vi "Single Loop QSM.vi"   [LabVIEW 2016, in "SLL QSM.lvlib"]
doc: "General Purpose Queue Based State Machine for Any Use Case (main application, module, pop up message etc)\n\n<b>Advantages:</b>\n1. No Need to Pass Queue References between Queue Driver VIs.\n2. This template can be safely used in multiple parallel running modules without any issues.\n3. This template can also be safely used even in cases where the VI is configured to be a Clone, where multiple \ninstances of the VI could be executing concurrently.\n\n<b>How to Use:</b>\n1. Add necessary items to the Main Cluster.\n2. Use the Polymorphic Queue Driver for doing any queue operations. There is no need to pass the queue driver\nreference, as the Queue Driver automatically infers the reference based on the VI instance from which it is called.\n3. Add any required user events in the \"Register Events\" case. Ignore if not needed.\n4. Use \"Sequences\" section for defining any list of state calls, which could be used in multiple places. \nEg: Initialize Sequence, might be needed if we need to any reinitialization."
uses:
  SLL QSM.lvlib
  <vilib>/Utility/error.llb/DialogType.ctl
  Queue Driver/Create Queue.vi
  Queue Driver/Enqueue an Item to Queue.vi
  Queue Driver/Dequeue Queue.vi
  Queue Driver/Enqueue N Items.vi
  Queue Driver/Flush Queue.vi
  Queue Driver/Release Queue.vi
types:
  T1 = typedef "DialogType.ctl" = u16
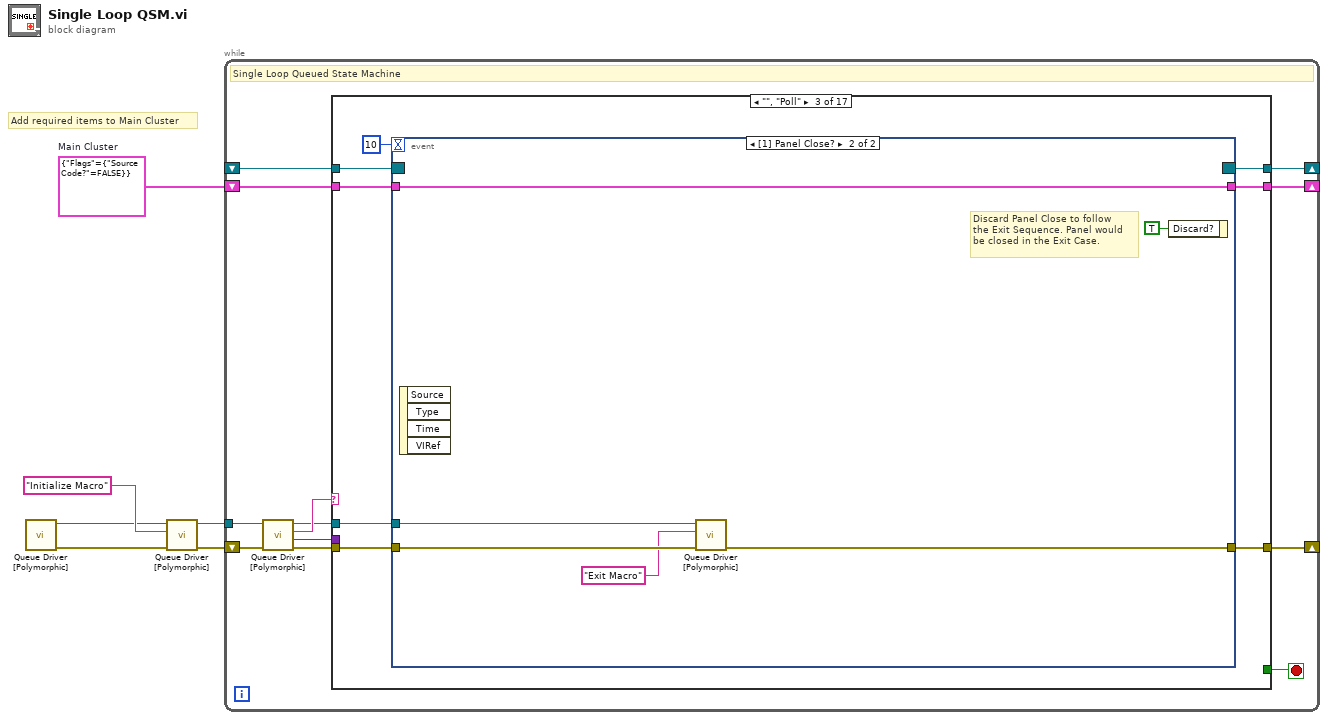
[diagram p0: block diagram]
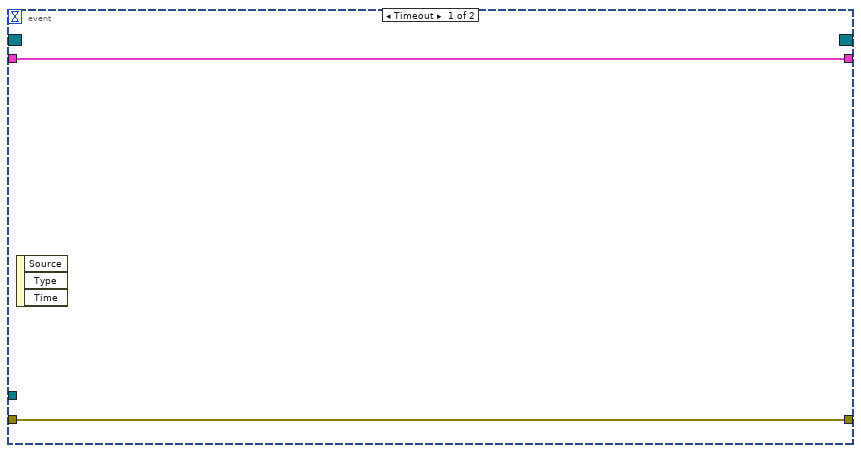
[diagram p4: hidden frame]
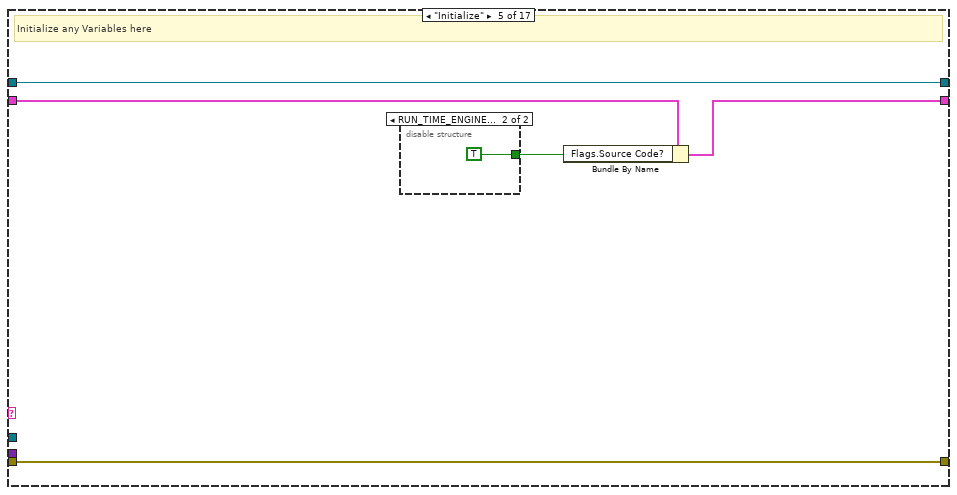
[diagram p6: hidden frame]
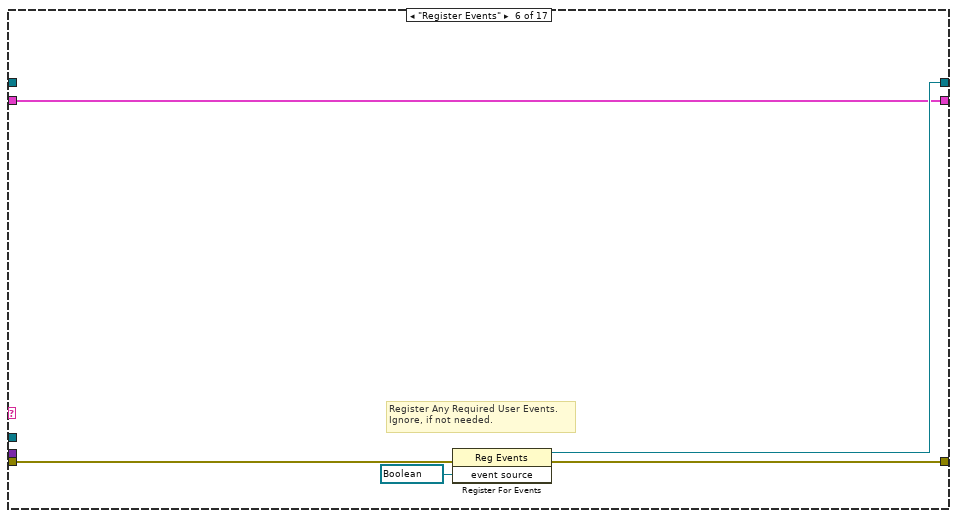
[diagram p8: hidden frame]
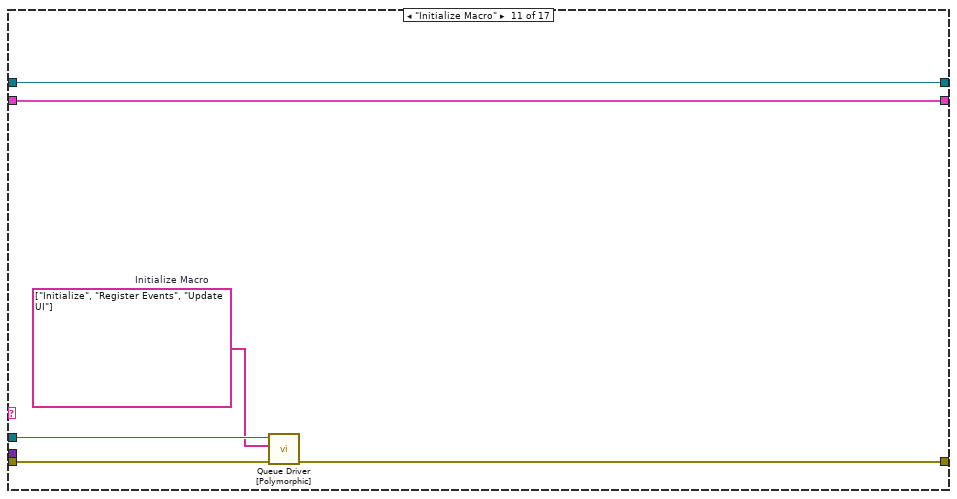
[diagram p13: hidden frame]
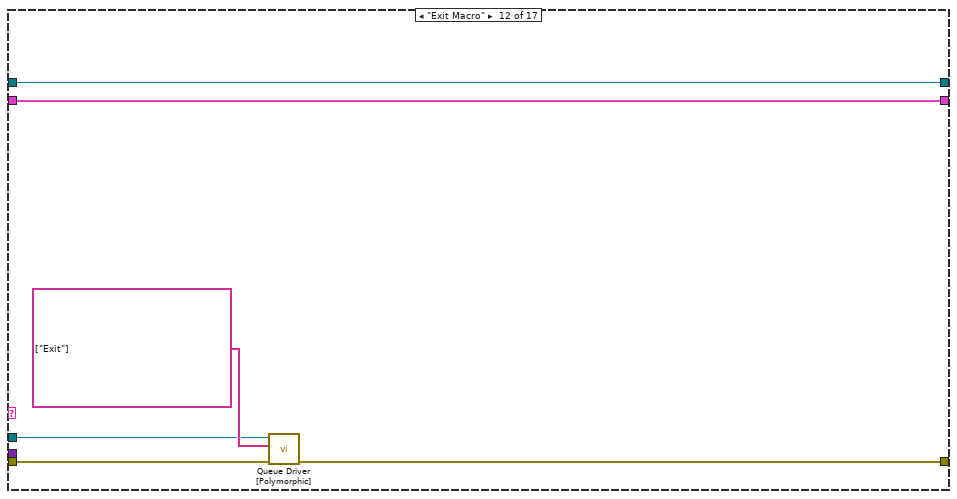
[diagram p14: hidden frame]
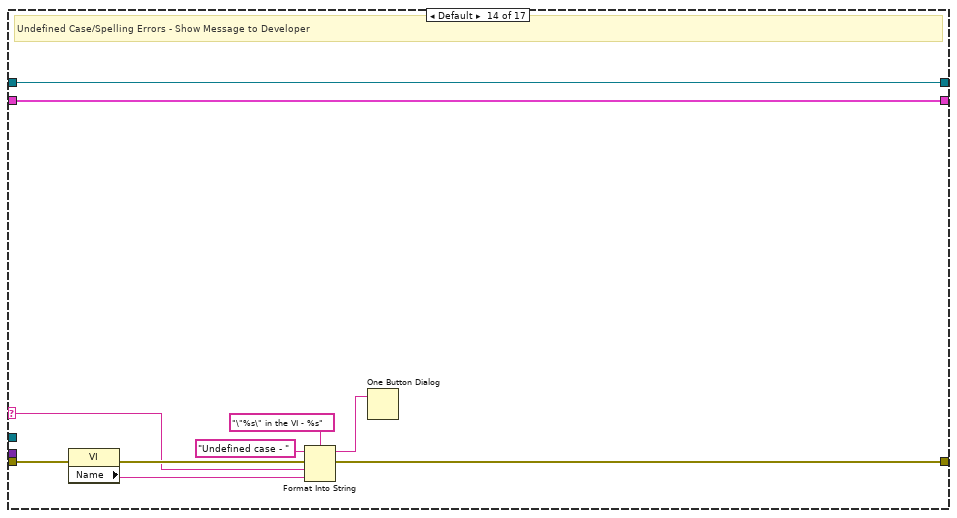
[diagram p16: hidden frame]
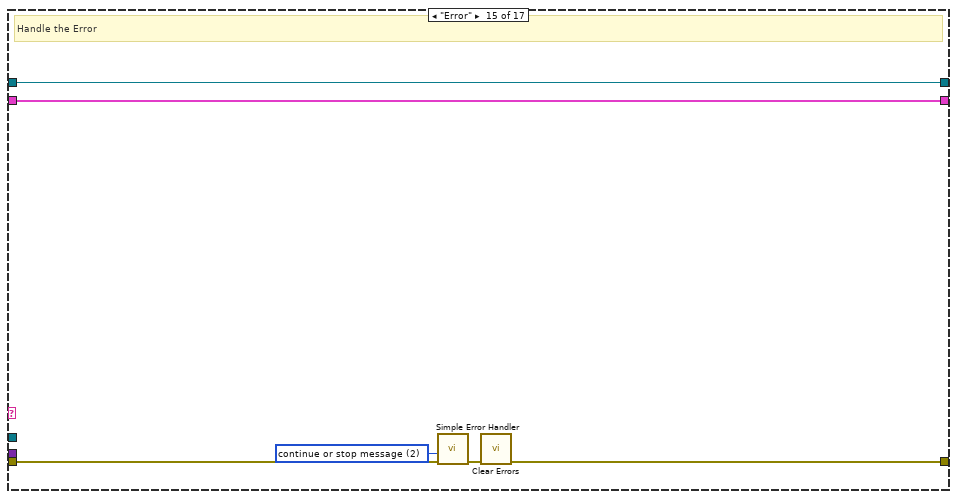
[diagram p17: hidden frame]
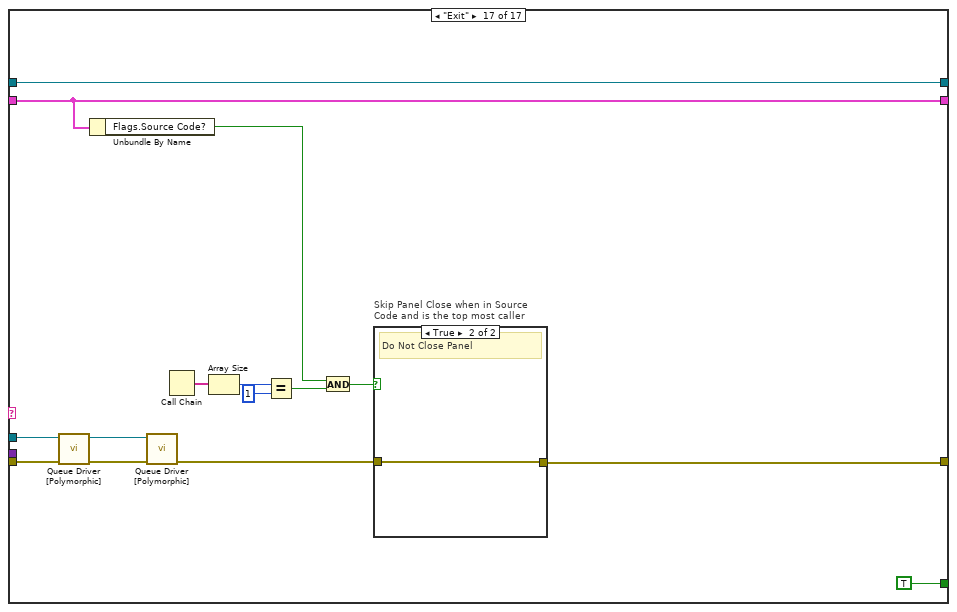
[diagram p19: hidden frame]
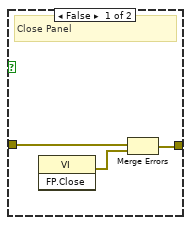
[diagram p20: hidden frame]
diagram:
  w4 = cluster{"Flags":cluster{"Source Code?":bool}} {"Flags"={"Source Code?"=FALSE}}  # Main Cluster
  # "Add required items to Main Cluster"
  n1 = call-poly "Queue Driver [Polymorphic].vi"() -> ("Error Out"=w6:errorcluster, "Queue Ref"=w2:refnum<queue>)  [unwired: 10 in]
  n2 = call-poly "Queue Driver [Polymorphic].vi"("Error In"=w6, "Item to Add"="Initialize Macro", "Queue Ref In"=w2) -> ("Error Out"=w5:errorcluster, "Queue Ref Out"=w1:refnum<queue>)  [unwired: 7 in]
  n3 = while "SLL Queued State Machine" {
    shift-right: [w16] -> _
    shift-left: w5 -> [w18]
    shift-right: [w14] -> _
    shift-left: _ -> [w13]
    shift-right: [w12] -> _
    shift-left: w4 -> [w11]
    tunnel: w1 -> [w9]
    stop <- w15 stop-if-true
    # "Single Loop Queued State Machine"
    n4 = call-poly "Queue Driver [Polymorphic].vi"("Error In"=w18, "Queue Ref In"=w9) -> ("Error Out"=w17:errorcluster, "Data"=w7:variant, "Dequeue"=w10:string, "Queue Ref Out"=w8:refnum<queue>)  [unwired: 6 in]
    n5 = case "QSM Case Structure" shown="\"\", \"Poll\"" w10 {
      selector: w10 -> [_ _ _ _ _ _ _ _ _ _ _ _ _ w82 _ _ _]
      tunnel: w17 -> [w21 w24 w30 w43 w48 w54 w57 w60 w63 w66 w70 w76 w81 w85 w97 w100 w113]
      tunnel: [w21 w24 w31 w43 w48 w53 w57 w60 w63 w66 w69 w75 w81 w88 w95 w100 w109] -> w16
      tunnel: [_ _ _ _ _ _ _ _ _ _ _ _ _ _ _ _ TRUE] -> w15
      tunnel: [w20 w23 w29 w42 w47 w52 w56 w59 w62 w65 w72 w78 w80 w91 w94 w99 w112] -> w14
      tunnel: w13 -> [w20 w23 w28 w42 w47 _ w56 w59 w62 w65 w72 w78 w80 w91 w94 w99 w112]
      tunnel: [w19 w22 w26 w41 w44 w51 w55 w58 w61 w64 w71 w77 w79 w90 w93 w98 w111] -> w12
      tunnel: w11 -> [w19 w22 w27 w41 w45 w51 w55 w58 w61 w64 w71 w77 w79 w90 w93 w98 w111]
      tunnel: w8 -> [_ _ w25 _ _ _ _ _ _ _ w68 w73 _ _ _ _ w102]
      tunnel: w7 -> [_ _ _ _ _ _ _ _ _ _ _ _ _ _ _ _ _]
      frame "/--------------- Read Me -----------------/" {
        # "General Purpose Queue Based State Machine for Any Use Case (main application, module, pop up message etc)\n\nAdvantages:\n1. No Need to Pass Queue References between Queue Driver VIs.\n2. This template can be safely used in multiple parallel running modules without any issues.\n3. This template can also be safely used even in cases where the VI is configured to be a Clone, where multiple \ninstances of the VI could be executing concurrently.\n\nHow to Use:\n1. Add necessary items to the Main Cluster.\n2. Use the Polymorphic Queue Driver for doing any queue operations. There is no need to pass the queue driver\nreference, as the Queue Driver automatically infers the reference based on the VI instance from which it is called.\n3. Add any required user events in the \"Register Events\" case. Ignore if not needed.\n4. Use \"Sequences\" section for defining any list of state calls, which could be used in multiple places. \nEg: Initialize Sequence, might be needed if we need to any reinitialization."
      }
      frame "/------------------ Poll -------------------/" {
      }
      frame "", "Poll" {
        n6 = event shown="[1] Panel Close?" {
          selector: w28 -> [_ _]
          dyn-events: [_ _] -> w29
          timeout: 10 -> [_ _]
          tunnel: [w34 w39] -> w31
          tunnel: w30 -> [w34 w40]
          tunnel: w27 -> [w33 w38]
          tunnel: [w33 w38] -> w26
          tunnel: w25 -> [_ w36]
          event Timeout {
            n7 = event-data() -> ()  [unwired: 1 in, 3 out]
          }
          event Panel Close? {
            # "Discard Panel Close to follow\nthe Exit Sequence. Panel would\nbe closed in the Exit Case."
            n8 = event-data() -> ()  [unwired: 1 in, 4 out]
            n9 = call-poly "Queue Driver [Polymorphic].vi"("Error In"=w40, "Item to Add"="Exit Macro" ("Enqueue"), "Queue Ref In"=w36) -> ("Error Out"=w39:errorcluster)  [unwired: 7 in, 1 out]
            n10 = event-data("Discard?"=TRUE) -> ()  [unwired: 1 in, 1 out]
          }
        }
      }
      frame "/--------------- Initialize -----------------/" {
      }
      frame "Initialize" {
        # "Initialize any Variables here"
        n11 = disable-structure shown="RUN_TIME_ENGINE==False" {
          disable-tunnel: [_ TRUE] -> w46
          frame condition #0 {
          }
          frame condition #1 (active) {
          }
        }
        n12 = Bundle By Name(cluster=w45, "Flags.Source Code?"=w46) -> (w44:cluster{"Flags":cluster{"Source Code?":bool}})
      }
      frame "Register Events" {
        # "Register Any Required User Events. \nIgnore, if not needed."
        n13 = register-events(error in=w54, refnum<vi> refnum ("event source")) -> (reference out=w52:refnum<event-registration>, error out=w53:errorcluster)  [unwired: 1 in]
      }
      frame "/---------- Custom Case Splitter ----------/" {
      }
      frame "/-------------- User Interface --------------/" {
        # "Duplicate this case to create additional case splitters for readability"
      }
      frame "Update UI" {
        # "Update Front Panel Controls in this Case"
      }
      frame "/----------------- Macros -----------------/" {
      }
      frame "Initialize Macro" {
        w67 = string[] ["Initialize", "Register Events", "Update UI"]  # Initialize Macro
        n14 = call-poly "Queue Driver [Polymorphic].vi"("Error In"=w70, "Enqueue N"=w67, "Queue Ref In"=w68) -> ("Error Out"=w69:errorcluster)  [unwired: 7 in, 1 out]
      }
      frame "Exit Macro" {
        n15 = call-poly "Queue Driver [Polymorphic].vi"("Error In"=w76, "Enqueue N"=string[] ["Exit"], "Queue Ref In"=w73) -> ("Error Out"=w75:errorcluster)  [unwired: 7 in, 1 out]
      }
      frame "/-------------- Error Handler--------------/" {
      }
      frame Default {
        # "Undefined Case/Spelling Errors - Show Message to Developer"
        n16 = property class="VI"(error in=w85) -> (error out=w84:errorcluster, "Name"=w83:string)  [unwired: 1 in, 1 out]
        n17 = Format Into String(format string="\"%s\" in the VI - %s" ("message"), initial string="Undefined case - ", error in=w84, w82, w83) -> (resulting string=w86:string, error out=w88:errorcluster)
        n18 = One Button Dialog(message=w86) -> ()  [unwired: 1 in, 1 out]
      }
      frame "Error" {
        w92 = T1 2 items=["no dialog", "OK message", "continue or stop message", "OK message + warnings", "continue/stop + warnings"] ("type of dialog (OK msg:1)")
        # "Handle the Error"
        n19 = call <vilib>:"Simple Error Handler.vi"("type of dialog (OK msg:1)"=w92, "error in (no error)"=w97) -> ("error out"=w96:errorcluster)  [unwired: 3 in, 4 out]
        n20 = call <vilib>:"Clear Errors.vi"("error in (no error)"=w96) -> ("error out"=w95:errorcluster)  [unwired: 5 in, 1 out]
      }
      frame "/------------------- Exit --------------------/" {
      }
      frame "Exit" {
        n21 = call-poly "Queue Driver [Polymorphic].vi"("Error In"=w113, "Queue Ref In"=w102) -> ("Error Out"=w114:errorcluster, "Queue Ref Out"=w101:refnum<queue>)  [unwired: 7 in, 1 out]
        n22 = Unbundle By Name(w111) -> ("Flags.Source Code?"=w104:bool)
        n23 = call-poly "Queue Driver [Polymorphic].vi"("Error In"=w114, "Queue Ref In"=w101) -> ("Error Out"=w110:errorcluster)  [unwired: 9 in]
        n24 = Call Chain() -> (call chain=w108:string[])
        n25 = Array Size(array=w108) -> (size(s)=w107:i32)
        n26 = Equal?(x=w107, y=1) -> (x = y?=w105:bool)
        n27 = And(x=w104, y=w105) -> (x .and. y?=w103:bool)
        n28 = case "Skip Panel Close when in Source\nCode and is the top most caller" shown="True" w103 {
          tunnel: w110 -> [w117 w119]
          tunnel: [w118 w119] -> w109
          frame False {
            # "Close Panel"
            n29 = invoke class="VI" method="FP.Close"() -> (error out=w116:errorcluster)  [unwired: 3 in, 2 out]
            n30 = Merge Errors(w117, w116) -> (w118:errorcluster)
          }
          frame True {
            # "Do Not Close Panel"
          }
        }
      }
    }
  }
